vi "setBrush.vi"(7 "colorGroup (All)":T2=5 items=["Active"=0, "Disabled"=1, "Inactive"=2, "All"=5], 8 "Error In":errorcluster, 9 "brush":refnum<class "QBrush.lvclass">, 10 "colorRole (NoRole)":T1=17 items=["WindowText", "Button", "Light", "Midlight", "Dark", "Mid", "Text", "BrightText", "ButtonText", "Base", "Window", "Shadow", "Highlight", "HighlightedText", "Link", "LinkVisited", "AlternateBase", "NoRole", "ToolTipBase", "ToolTipText", "PlaceholderText"], 11 "QPalette In":refnum<class "QPalette.lvclass">) -> (0 "Error Out":errorcluster, 3 "QPalette Out":refnum<class "QPalette.lvclass">)   [LabVIEW 2014, in "QPalette.lvclass"]
doc: "LabVIEW-specific documentation is not yet available. See <b>https://doc.qt.io/qt-5/qpalette.html#setBrush</b>"
uses:
  QPalette.lvclass
  ColorGroup.ctl
  ColorRole.ctl
  QBrush/QBrush.lvclass
  LQ Core/LQSerialData/LQSerialData.lvclass/LQSerialData.ctl
  LQ Core/LQ Core.lvlib
  LQ Core/LQSerialData/LQSerialData.lvclass
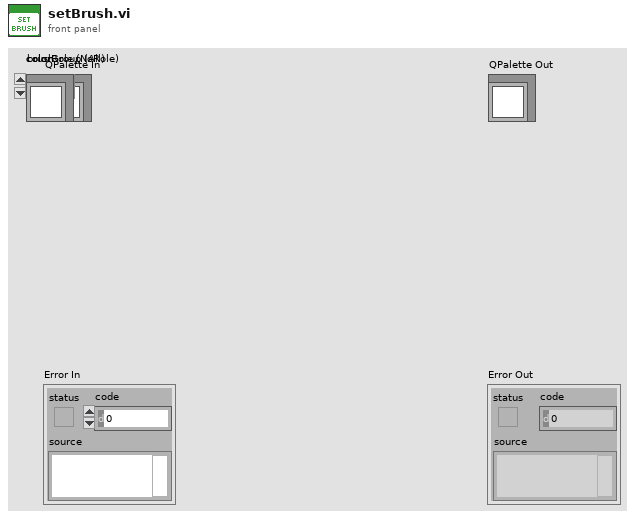
[diagram p1: front panel]
types:
  T1 = typedef "QPalette.lvclass/ColorRole.ctl" = i32
  T2 = typedef "QPalette.lvclass/ColorGroup.ctl" = i32
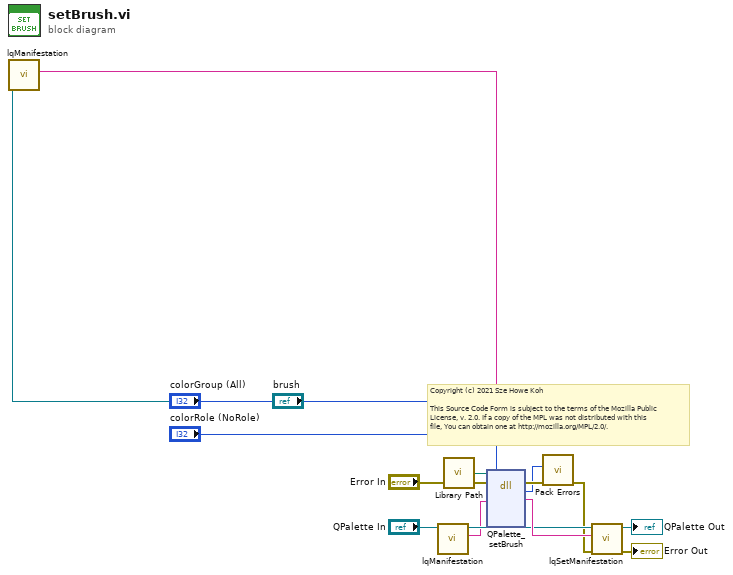
[diagram p0: block diagram]
diagram:
  # "Copyright (c) 2021 Sze Howe Koh\n\nThis Source Code Form is subject to the terms of the Mozilla Public\nLicense, v. 2.0. If a copy of the MPL was not distributed with this\nfile, You can obtain one at http://mozilla.org/MPL/2.0/."
  n1 = call "lqManifestation.vi"("LQSerialData in"="brush") -> ("Manifestation"=w1:string)  [unwired: 9 in, 1 out]
  n2 = call "lqManifestation.vi"("LQSerialData in"="QPalette In") -> ("Manifestation"=w10:string, "LQSerialData out"=w11:refnum<class "QPalette.lvclass">)  [unwired: 9 in]
  n3 = call "Library Path.vi"() -> ("Library Path"=w9:path)
  n4 = dll-call lib="?" fn="QPalette_setBrush"(path in=w9, error in="Error In", "_instance"=w10, "colorGroup"="colorGroup (All)", "colorRole"="colorRole (NoRole)", "brush"=w1) -> (error out=w8:errorcluster, w7:i32, "_instance"=w13:string)  [unwired: 4 in, 1 out]
  n5 = call "Pack Errors.vi"("Error In"=w8, "Error Code"=w7) -> ("Error Out"=w6:errorcluster)  [unwired: 9 in]
  n6 = call "lqSetManifestation.vi"("Error In"=w6, "Manifestation"=w13, "LQSerialData in"=w11) -> ("Error Out"=→"Error Out":errorcluster, "LQSerialData out"=→"QPalette Out":refnum<class "QPalette.lvclass">)  [unwired: 7 in]
